vi "Generate Landmark Array.vi"(6 "Observed LM Array":T1(array[cluster]), 8 "error in (no error)":errorcluster, 10 "SLAM In":T2) -> (0 "error out":errorcluster, 2 "SLAM Out":T2)   [LabVIEW 2009]
uses:
  Controls/SLAM.ctl
  <vilib>/Analysis/Matrix/Datatypes/RealMatrix.ctl
  <vilib>/Analysis/baseanly.llb/Real A x B.vi
  <vilib>/Analysis/Matrix/NI_Matrix.lvlib
  <vilib>/Analysis/NI_AALBase.lvlib
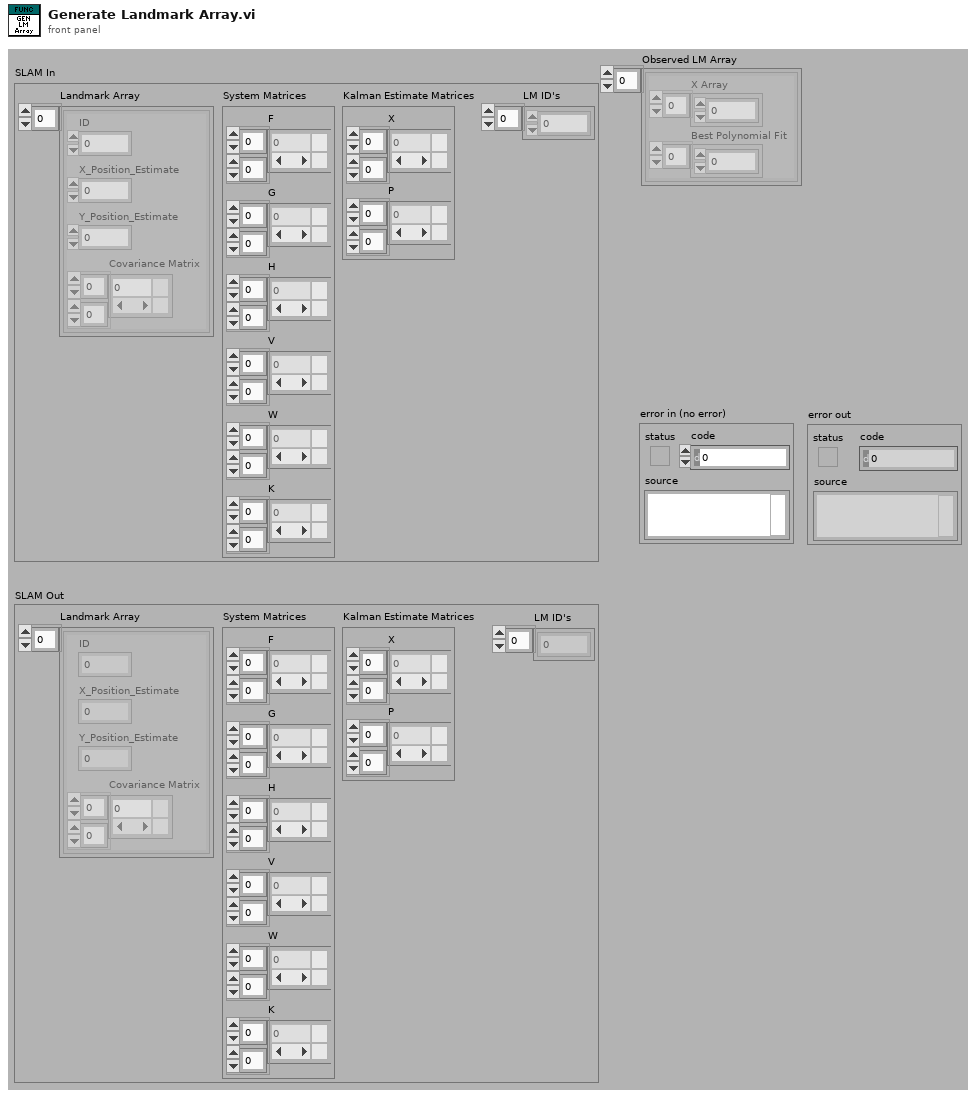
[diagram p1: front panel]
types:
  T1 = cluster{"X Array":dbl[], "Best Polynomial Fit":dbl[]}[]
  T2 = typedef "SLAM.ctl" = cluster{"Landmark Array":cluster{"ID":dbl, "X_Position_Estimate":dbl, "Y_Position_Estimate":dbl, "Covariance Matrix":T3}[], "System Matrices":cluster{"F":T3, "G":T3, "H":T3, "V":T3, "W":T3, "K":T3}, "Kalman Estimate Matrices":cluster{"X":T3, "P":T3}, "LM ID's":dbl[]}
  T3 = typedef "NI_Matrix.lvlib/RealMatrix.ctl" = dbl[][]
  T4 = cluster{"ID":dbl, "X_Position_Estimate":dbl, "Y_Position_Estimate":dbl, "Covariance Matrix":T3}[]
  T5 = cluster{"ID":dbl, "X_Position_Estimate":dbl, "Y_Position_Estimate":dbl, "Covariance Matrix":T3}
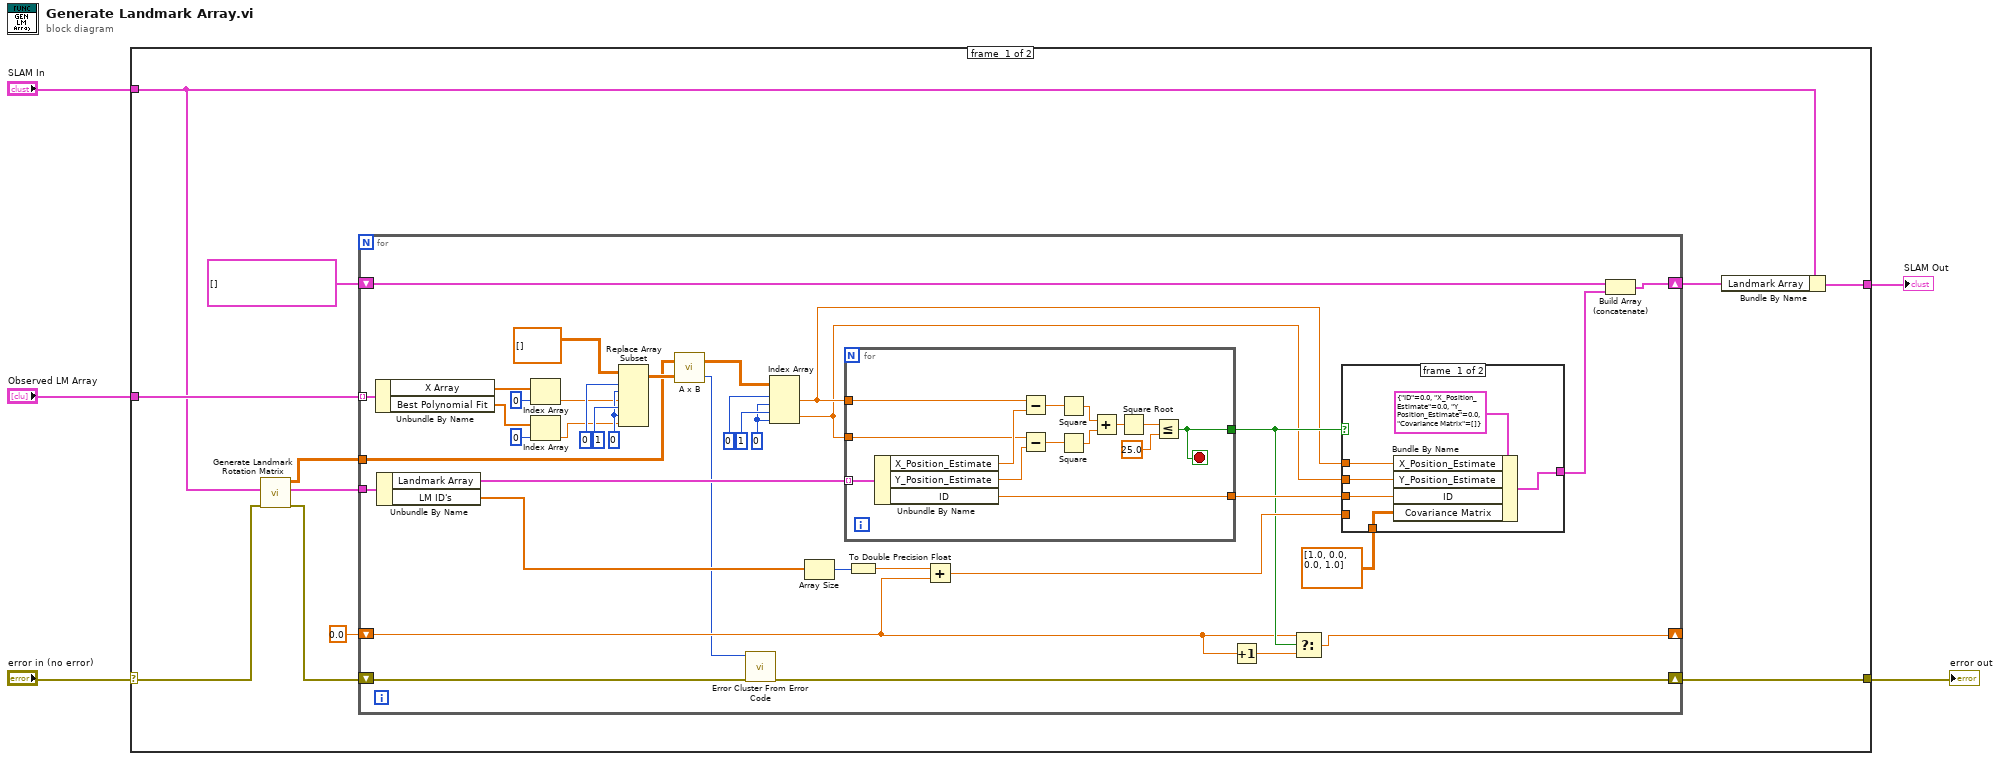
[diagram p0: block diagram]
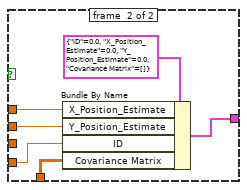
[diagram p2: hidden frame]
diagram:
  n1 = case shown="No Error" "error in (no error)" {
    selector: "error in (no error)" -> [w9 w80]
    tunnel: "SLAM In" -> [w11 w81]
    tunnel: [w16 w81] -> w4
    tunnel: "Observed LM Array" -> [w14 _]
    tunnel: [w6 w80] -> w1
    frame #0 {
      n2 = call "Generate Landmark Rotation Matrix.vi"("error in (no error)"=w9, "SLAM In"=w11) -> ("error out"=w7:errorcluster, "SLAM Out"=w10:T2, "Rotation matrix"=w8:T3)  [unwired: 7 in]
      n3 = for {
        tunnel: w14 -> [w42] mode=indexing
        shift-right: [w51] -> w13
        shift-left: T4 [] ("appended array") -> [w53]
        tunnel: w10 -> [w49]
        shift-right: [w34] -> _
        shift-left: 0.0 ("double precision float") -> [w35]
        tunnel: w8 -> [w26]
        shift-right: [w19] -> w6
        shift-left: w7 -> [w20]
        w23 = 0 ("index (col)")
        w30 = 0 ("index (col)")
        n4 = Unbundle By Name(w42) -> ("X Array"=w45:dbl[], "Best Polynomial Fit"=w46:dbl[])
        n5 = Unbundle By Name(w49) -> ("Landmark Array"=w50:T4, "LM ID's"=w48:dbl[])
        n6 = Index Array(array=w45, index=0) -> (element=w28:dbl)
        n7 = Index Array(array=w46, index=0) -> (element=w27:dbl)
        n8 = Replace Array Subset(array=T3 [] ("matrix"), new element #1=w28, index (row) #1=0 ("index (col)"), index (col) #1=w30, new element #2=w27, index (row) #2=1 ("index (col)"), index (col) #2=w30) -> (w33:T3)
        n9 = call-poly <vilib>:"A x B.vi"("B"=w33, "A"=w26) -> ("error"=w21:i32, "A x B"=w22:T3)
        n10 = call <vilib>:"Error Cluster From Error Code.vi"("error in (no error)"=w20, "error code (0)"=w21) -> ("error out"=w19:errorcluster)  [unwired: 7 in]
        n11 = Index Array(array=w22, index (row) #1=0 ("index (col)"), index (col) #1=w23, index (row) #2=1 ("index (col)"), index (col) #2=w23) -> (element #1=w18:dbl, element #2=w17:dbl)
        n12 = Array Size(array=w48) -> (size(s)=w40:i32)
        n13 = for {
          tunnel: w50 -> [w79] mode=indexing
          tunnel: [w69] -> w37
          tunnel: [w68] -> w47
          tunnel: w18 -> [w67]
          tunnel: w17 -> [w66]
          stop <- w69 stop-if-true
          n14 = Unbundle By Name(w79) -> ("X_Position_Estimate"=w71:dbl, "Y_Position_Estimate"=w70:dbl, "ID"=w68:dbl)
          n15 = Subtract(x=w67, y=w71) -> (x-y=w77:dbl)
          n16 = Subtract(x=w66, y=w70) -> (x-y=w78:dbl)
          n17 = Square(x=w77) -> (x^2=w76:dbl)
          n18 = Square(x=w78) -> (x^2=w75:dbl)
          n19 = Add(x=w76, y=w75) -> (x+y=w74:dbl)
          n20 = Square Root(x=w74) -> (sqrt(x)=w73:dbl)
          n21 = Less Or Equal?(x=w73, y=25.0) -> (x <= y?=w69:bool)
        }
        n22 = To Double Precision Float(number=w40) -> (double precision float=w39:dbl)
        n23 = Add(x=w39, y=w35) -> (x+y=w38:dbl)
        n24 = Increment(x=w35) -> (x+1=w36:dbl)
        n25 = Select(t=w35, s=w37, f=w36) -> (s? t:f=w34:dbl)
        n26 = case shown="False" w37 {
          tunnel: [w58 w64] -> w52
          tunnel: w47 -> [w57 _]
          tunnel: T3 [[1.0, 0.0], [0.0, 1.0]] ("Covariance Matrix") -> [w56 w63]
          tunnel: w38 -> [_ w62]
          tunnel: w18 -> [w55 w61]
          tunnel: w17 -> [w54 w60]
          frame #0 {
            n27 = Bundle By Name(cluster=T5 {"ID"=0.0, "X_Position_Estimate"=0.0, "Y_Position_Estimate"=0.0, "Covariance Matrix"=[]} ("Landmarks"), "X_Position_Estimate"=w55, "Y_Position_Estimate"=w54, "ID"=w57, "Covariance Matrix"=w56) -> (w58:T5)
          }
          frame #1 {
            n28 = Bundle By Name(cluster=T5 {"ID"=0.0, "X_Position_Estimate"=0.0, "Y_Position_Estimate"=0.0, "Covariance Matrix"=[]} ("Landmarks"), "X_Position_Estimate"=w61, "Y_Position_Estimate"=w60, "ID"=w62, "Covariance Matrix"=w63) -> (w64:T5)
          }
        }
        n29 = Build Array (concatenate)(w53, w52) -> (w51:T4)
      }
      n30 = Bundle By Name(cluster=w11, "Landmark Array"=w13) -> (w16:T2)
    }
    frame #1 {
    }
  }
  "SLAM Out" <- w4
  "error out" <- w1
